vi "PlotTrucks.vi"(1 "Trucks":T1, 2 "Lanes":T2) -> (0 "Truck positions":cluster{"X":dbl[], "Y":dbl[]}[](graph))   [LabVIEW 2013]
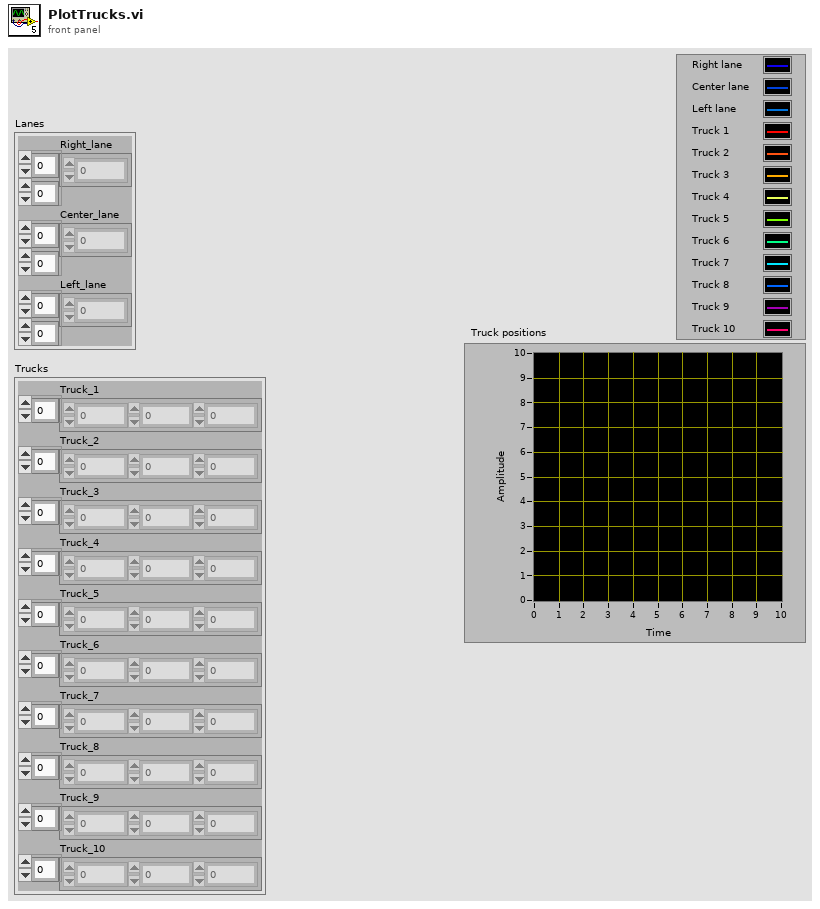
[diagram p1: front panel]
types:
  T1 = cluster{"Truck_1":dbl[], "Truck_2":dbl[], "Truck_3":dbl[], "Truck_4":dbl[], "Truck_5":dbl[], "Truck_6":dbl[], "Truck_7":dbl[], "Truck_8":dbl[], "Truck_9":dbl[], "Truck_10":dbl[]}
  T2 = cluster{"Right_lane":dbl[][], "Center_lane":dbl[][], "Left_lane":dbl[][]}
  T3 = cluster{"Truck_1[0]":dbl, "Truck_1[1]":dbl, "Truck_1[2]":dbl, "Truck_1[3]":dbl, "Truck_1[4]":dbl, "Truck_1[5]":dbl, "Truck_1[6]":dbl, "Truck_1[7]":dbl, "Truck_1[8]":dbl}
  T4 = cluster{"Truck_2[0]":dbl, "Truck_2[1]":dbl, "Truck_2[2]":dbl, "Truck_2[3]":dbl, "Truck_2[4]":dbl, "Truck_2[5]":dbl, "Truck_2[6]":dbl, "Truck_2[7]":dbl, "Truck_2[8]":dbl}
  T5 = cluster{"Truck_3[0]":dbl, "Truck_3[1]":dbl, "Truck_3[2]":dbl, "Truck_3[3]":dbl, "Truck_3[4]":dbl, "Truck_3[5]":dbl, "Truck_3[6]":dbl, "Truck_3[7]":dbl, "Truck_3[8]":dbl}
  T6 = cluster{"Truck_4[0]":dbl, "Truck_4[1]":dbl, "Truck_4[2]":dbl, "Truck_4[3]":dbl, "Truck_4[4]":dbl, "Truck_4[5]":dbl, "Truck_4[6]":dbl, "Truck_4[7]":dbl, "Truck_4[8]":dbl}
  T7 = cluster{"Truck_5[0]":dbl, "Truck_5[1]":dbl, "Truck_5[2]":dbl, "Truck_5[3]":dbl, "Truck_5[4]":dbl, "Truck_5[5]":dbl, "Truck_5[6]":dbl, "Truck_5[7]":dbl, "Truck_5[8]":dbl}
  T8 = cluster{"Truck_6[0]":dbl, "Truck_6[1]":dbl, "Truck_6[2]":dbl, "Truck_6[3]":dbl, "Truck_6[4]":dbl, "Truck_6[5]":dbl, "Truck_6[6]":dbl, "Truck_6[7]":dbl, "Truck_6[8]":dbl}
  T9 = cluster{"Truck_7[0]":dbl, "Truck_7[1]":dbl, "Truck_7[2]":dbl, "Truck_7[3]":dbl, "Truck_7[4]":dbl, "Truck_7[5]":dbl, "Truck_7[6]":dbl, "Truck_7[7]":dbl, "Truck_7[8]":dbl}
  T10 = cluster{"Truck_8[0]":dbl, "Truck_8[1]":dbl, "Truck_8[2]":dbl, "Truck_8[3]":dbl, "Truck_8[4]":dbl, "Truck_8[5]":dbl, "Truck_8[6]":dbl, "Truck_8[7]":dbl, "Truck_8[8]":dbl}
  T11 = cluster{"Truck_9[0]":dbl, "Truck_9[1]":dbl, "Truck_9[2]":dbl, "Truck_9[3]":dbl, "Truck_9[4]":dbl, "Truck_9[5]":dbl, "Truck_9[6]":dbl, "Truck_9[7]":dbl, "Truck_9[8]":dbl}
  T12 = cluster{"Truck_10[0]":dbl, "Truck_10[1]":dbl, "Truck_10[2]":dbl, "Truck_10[3]":dbl, "Truck_10[4]":dbl, "Truck_10[5]":dbl, "Truck_10[6]":dbl, "Truck_10[7]":dbl, "Truck_10[8]":dbl}
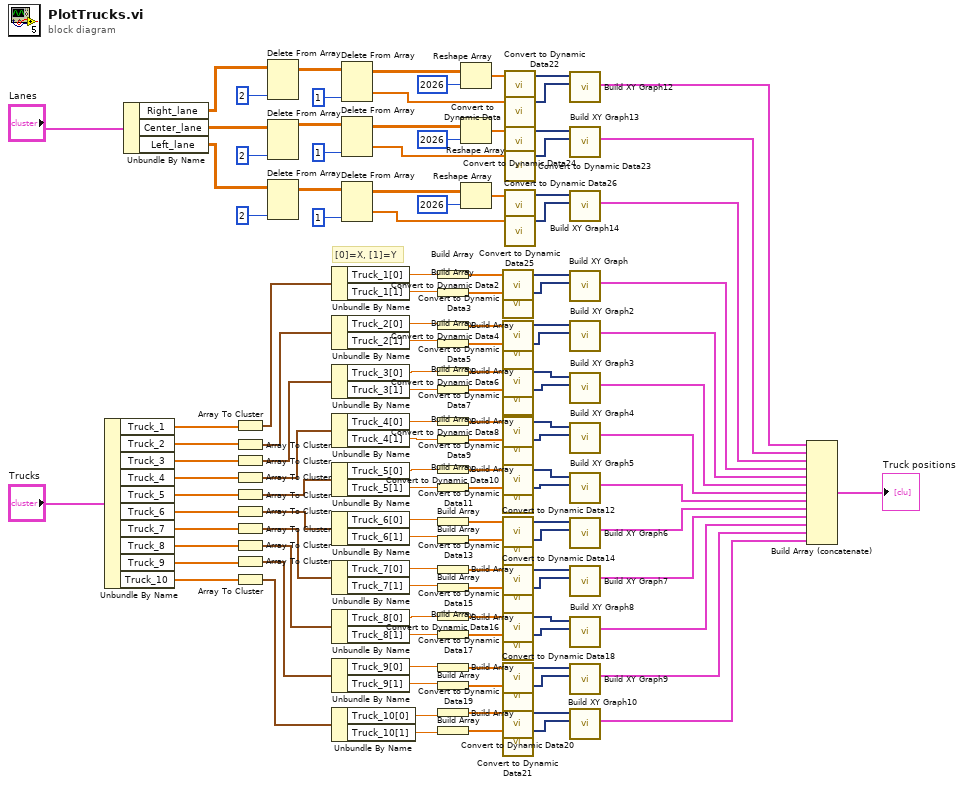
[diagram p0: block diagram]
diagram:
  # "[0]=X, [1]=Y"
  n1 = Unbundle By Name("Trucks") -> ("Truck_1"=w125:dbl[], "Truck_2"=w123:dbl[], "Truck_3"=w122:dbl[], "Truck_4"=w121:dbl[], "Truck_5"=w120:dbl[], "Truck_6"=w119:dbl[], "Truck_7"=w118:dbl[], "Truck_8"=w117:dbl[], "Truck_9"=w116:dbl[], "Truck_10"=w115:dbl[])
  n2 = Unbundle By Name("Lanes") -> ("Right_lane"=w34:dbl[][], "Center_lane"=w29:dbl[][], "Left_lane"=w30:dbl[][])
  n3 = Array To Cluster(array=w125) -> (cluster=w124:T3)
  n4 = Array To Cluster(array=w123) -> (cluster=w114:T4)
  n5 = Array To Cluster(array=w122) -> (cluster=w113:T5)
  n6 = Array To Cluster(array=w121) -> (cluster=w112:T6)
  n7 = Array To Cluster(array=w120) -> (cluster=w111:T7)
  n8 = Array To Cluster(array=w119) -> (cluster=w110:T8)
  n9 = Array To Cluster(array=w118) -> (cluster=w109:T9)
  n10 = Array To Cluster(array=w117) -> (cluster=w108:T10)
  n11 = Array To Cluster(array=w116) -> (cluster=w107:T11)
  n12 = Array To Cluster(array=w115) -> (cluster=w106:T12)
  n13 = Delete From Array(array=w34, index (col)=2 ("disabled index (col)")) -> (array with subset deleted=w23:dbl[][])  [unwired: 2 in, 1 out]
  n14 = Delete From Array(array=w29, index (col)=2 ("disabled index (col)")) -> (array with subset deleted=w24:dbl[][])  [unwired: 2 in, 1 out]
  n15 = Delete From Array(array=w30, index (col)=2 ("disabled index (col)")) -> (array with subset deleted=w25:dbl[][])  [unwired: 2 in, 1 out]
  n16 = Unbundle By Name(w124) -> ("Truck_1[0]"=w105:dbl, "Truck_1[1]"=w101:dbl)
  n17 = Unbundle By Name(w114) -> ("Truck_2[0]"=w63:dbl, "Truck_2[1]"=w62:dbl)
  n18 = Unbundle By Name(w113) -> ("Truck_3[0]"=w61:dbl, "Truck_3[1]"=w60:dbl)
  n19 = Unbundle By Name(w112) -> ("Truck_4[0]"=w59:dbl, "Truck_4[1]"=w58:dbl)
  n20 = Unbundle By Name(w111) -> ("Truck_5[0]"=w57:dbl, "Truck_5[1]"=w56:dbl)
  n21 = Unbundle By Name(w110) -> ("Truck_6[0]"=w55:dbl, "Truck_6[1]"=w54:dbl)
  n22 = Unbundle By Name(w109) -> ("Truck_7[0]"=w53:dbl, "Truck_7[1]"=w52:dbl)
  n23 = Unbundle By Name(w108) -> ("Truck_8[0]"=w51:dbl, "Truck_8[1]"=w50:dbl)
  n24 = Unbundle By Name(w107) -> ("Truck_9[0]"=w49:dbl, "Truck_9[1]"=w48:dbl)
  n25 = Unbundle By Name(w106) -> ("Truck_10[0]"=w47:dbl, "Truck_10[1]"=w46:dbl)
  n26 = Delete From Array(array=w23, index (col)=1 ("disabled index (col)")) -> (deleted portion=w5:dbl[], array with subset deleted=w16:dbl[][])  [unwired: 2 in]
  n27 = Delete From Array(array=w24, index (col)=1 ("disabled index (col)")) -> (deleted portion=w13:dbl[], array with subset deleted=w15:dbl[][])  [unwired: 2 in]
  n28 = Delete From Array(array=w25, index (col)=1 ("disabled index (col)")) -> (deleted portion=w11:dbl[], array with subset deleted=w14:dbl[][])  [unwired: 2 in]
  n29 = Build Array(w105) -> (w104:dbl[])
  n30 = Build Array(w101) -> (w102:dbl[])
  n31 = Build Array(w63) -> (w96:dbl[])
  n32 = Build Array(w62) -> (w98:dbl[])
  n33 = Build Array(w61) -> (w95:dbl[])
  n34 = Build Array(w60) -> (w93:dbl[])
  n35 = Build Array(w59) -> (w88:dbl[])
  n36 = Build Array(w58) -> (w90:dbl[])
  n37 = Build Array(w57) -> (w87:dbl[])
  n38 = Build Array(w56) -> (w85:dbl[])
  n39 = Build Array(w55) -> (w80:dbl[])
  n40 = Build Array(w54) -> (w82:dbl[])
  n41 = Build Array(w53) -> (w79:dbl[])
  n42 = Build Array(w52) -> (w77:dbl[])
  n43 = Build Array(w51) -> (w72:dbl[])
  n44 = Build Array(w50) -> (w74:dbl[])
  n45 = Build Array(w49) -> (w71:dbl[])
  n46 = Build Array(w48) -> (w69:dbl[])
  n47 = Build Array(w47) -> (w64:dbl[])
  n48 = Build Array(w46) -> (w66:dbl[])
  n49 = Reshape Array(w16, 2026 ("dimension size")) -> (w6:dbl[])
  n50 = Reshape Array(w15, 2026 ("dimension size")) -> (w12:dbl[])
  n51 = Reshape Array(w14, 2026 ("dimension size")) -> (w7:dbl[])
  n52 = call "Convert to Dynamic Data2"("Array"=w104) -> ("Dynamic Data Type"=w103:dynamicdata)  [unwired: 3 in]
  n53 = call "Convert to Dynamic Data3"("Array"=w102) -> ("Dynamic Data Type"=w100:dynamicdata)  [unwired: 3 in]
  n54 = call "Convert to Dynamic Data4"("Array"=w96) -> ("Dynamic Data Type"=w97:dynamicdata)  [unwired: 3 in]
  n55 = call "Convert to Dynamic Data5"("Array"=w98) -> ("Dynamic Data Type"=w99:dynamicdata)  [unwired: 3 in]
  n56 = call "Convert to Dynamic Data6"("Array"=w95) -> ("Dynamic Data Type"=w94:dynamicdata)  [unwired: 3 in]
  n57 = call "Convert to Dynamic Data7"("Array"=w93) -> ("Dynamic Data Type"=w92:dynamicdata)  [unwired: 3 in]
  n58 = call "Convert to Dynamic Data8"("Array"=w88) -> ("Dynamic Data Type"=w89:dynamicdata)  [unwired: 3 in]
  n59 = call "Convert to Dynamic Data9"("Array"=w90) -> ("Dynamic Data Type"=w91:dynamicdata)  [unwired: 3 in]
  n60 = call "Convert to Dynamic Data10"("Array"=w87) -> ("Dynamic Data Type"=w86:dynamicdata)  [unwired: 3 in]
  n61 = call "Convert to Dynamic Data11"("Array"=w85) -> ("Dynamic Data Type"=w84:dynamicdata)  [unwired: 3 in]
  n62 = call "Convert to Dynamic Data12"("Array"=w80) -> ("Dynamic Data Type"=w81:dynamicdata)  [unwired: 3 in]
  n63 = call "Convert to Dynamic Data13"("Array"=w82) -> ("Dynamic Data Type"=w83:dynamicdata)  [unwired: 3 in]
  n64 = call "Convert to Dynamic Data14"("Array"=w79) -> ("Dynamic Data Type"=w78:dynamicdata)  [unwired: 3 in]
  n65 = call "Convert to Dynamic Data15"("Array"=w77) -> ("Dynamic Data Type"=w76:dynamicdata)  [unwired: 3 in]
  n66 = call "Convert to Dynamic Data16"("Array"=w72) -> ("Dynamic Data Type"=w73:dynamicdata)  [unwired: 3 in]
  n67 = call "Convert to Dynamic Data17"("Array"=w74) -> ("Dynamic Data Type"=w75:dynamicdata)  [unwired: 3 in]
  n68 = call "Convert to Dynamic Data18"("Array"=w71) -> ("Dynamic Data Type"=w70:dynamicdata)  [unwired: 3 in]
  n69 = call "Convert to Dynamic Data19"("Array"=w69) -> ("Dynamic Data Type"=w68:dynamicdata)  [unwired: 3 in]
  n70 = call "Convert to Dynamic Data20"("Array"=w64) -> ("Dynamic Data Type"=w65:dynamicdata)  [unwired: 3 in]
  n71 = call "Convert to Dynamic Data21"("Array"=w66) -> ("Dynamic Data Type"=w67:dynamicdata)  [unwired: 3 in]
  n72 = call "Convert to Dynamic Data22"("Array"=w6) -> ("Dynamic Data Type"=w22:dynamicdata)  [unwired: 3 in]
  n73 = call "Convert to Dynamic Data"("Array"=w5) -> ("Dynamic Data Type"=w21:dynamicdata)  [unwired: 3 in]
  n74 = call "Convert to Dynamic Data24"("Array"=w12) -> ("Dynamic Data Type"=w19:dynamicdata)  [unwired: 3 in]
  n75 = call "Convert to Dynamic Data23"("Array"=w13) -> ("Dynamic Data Type"=w20:dynamicdata)  [unwired: 3 in]
  n76 = call "Convert to Dynamic Data26"("Array"=w7) -> ("Dynamic Data Type"=w18:dynamicdata)  [unwired: 3 in]
  n77 = call "Convert to Dynamic Data25"("Array"=w11) -> ("Dynamic Data Type"=w17:dynamicdata)  [unwired: 3 in]
  n78 = call "Build XY Graph12"("Y Input"=w21, "X Input"=w22) -> ("XY Graph"=w1:cluster{"X":dbl[], "Y":dbl[]}[])  [unwired: 8 in, 1 out]
  n79 = call "Build XY Graph13"("Y Input"=w20, "X Input"=w19) -> ("XY Graph"=w2:cluster{"X":dbl[], "Y":dbl[]}[])  [unwired: 8 in, 1 out]
  n80 = call "Build XY Graph14"("Y Input"=w17, "X Input"=w18) -> ("XY Graph"=w3:cluster{"X":dbl[], "Y":dbl[]}[])  [unwired: 8 in, 1 out]
  n81 = call "Build XY Graph"("Y Input"=w100, "X Input"=w103) -> ("XY Graph"=w45:cluster{"X":dbl[], "Y":dbl[]}[])  [unwired: 8 in, 1 out]
  n82 = call "Build XY Graph2"("Y Input"=w99, "X Input"=w97) -> ("XY Graph"=w44:cluster{"X":dbl[], "Y":dbl[]}[])  [unwired: 8 in, 1 out]
  n83 = call "Build XY Graph3"("Y Input"=w92, "X Input"=w94) -> ("XY Graph"=w42:cluster{"X":dbl[], "Y":dbl[]}[])  [unwired: 8 in, 1 out]
  n84 = call "Build XY Graph4"("Y Input"=w91, "X Input"=w89) -> ("XY Graph"=w41:cluster{"X":dbl[], "Y":dbl[]}[])  [unwired: 8 in, 1 out]
  n85 = call "Build XY Graph5"("Y Input"=w84, "X Input"=w86) -> ("XY Graph"=w40:cluster{"X":dbl[], "Y":dbl[]}[])  [unwired: 8 in, 1 out]
  n86 = call "Build XY Graph6"("Y Input"=w83, "X Input"=w81) -> ("XY Graph"=w39:cluster{"X":dbl[], "Y":dbl[]}[])  [unwired: 8 in, 1 out]
  n87 = call "Build XY Graph7"("Y Input"=w76, "X Input"=w78) -> ("XY Graph"=w38:cluster{"X":dbl[], "Y":dbl[]}[])  [unwired: 8 in, 1 out]
  n88 = call "Build XY Graph8"("Y Input"=w75, "X Input"=w73) -> ("XY Graph"=w37:cluster{"X":dbl[], "Y":dbl[]}[])  [unwired: 8 in, 1 out]
  n89 = call "Build XY Graph9"("Y Input"=w68, "X Input"=w70) -> ("XY Graph"=w36:cluster{"X":dbl[], "Y":dbl[]}[])  [unwired: 8 in, 1 out]
  n90 = call "Build XY Graph10"("Y Input"=w67, "X Input"=w65) -> ("XY Graph"=w35:cluster{"X":dbl[], "Y":dbl[]}[])  [unwired: 8 in, 1 out]
  n91 = Build Array (concatenate)(w1, w2, w3, w45, w44, w42, w41, w40, w39, w38, w37, w36, w35) -> (→"Truck positions":cluster{"X":dbl[], "Y":dbl[]}[])
